vi "GetParam.vi"(8 "error in (no error)":errorcluster caption="entrée d'erreur (pas d'erreur)", 11 "Balanced_Accuracy_Score.lvclass":refnum<class "Balanced_Accuracy_Score.lvclass">) -> (0 "error out":errorcluster caption="sortie d'erreur", 2 "balanced_accuracy_score":cluster{"sample_weight":dbl[], "adjusted":bool}, 3 "Balanced_Accuracy_Score.lvclass":refnum<class "Balanced_Accuracy_Score.lvclass">)   [LabVIEW 2020, in "Balanced_Accuracy_Score.lvclass"]
doc: "Get Parameters"
uses:
  Balanced_Accuracy_Score.lvclass
  Balanced_Accuracy_Score.lvclass/Balanced_Accuracy_Score.ctl
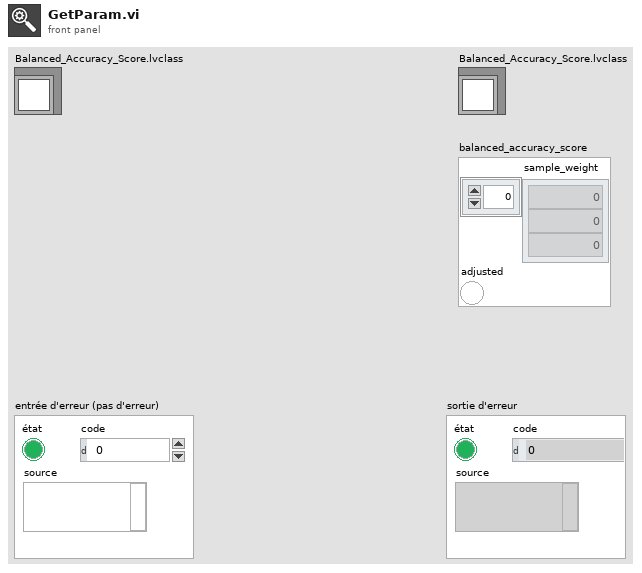
[diagram p1: front panel]
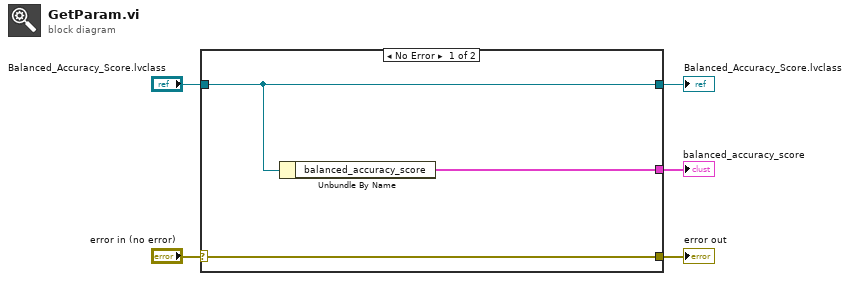
[diagram p0: block diagram]
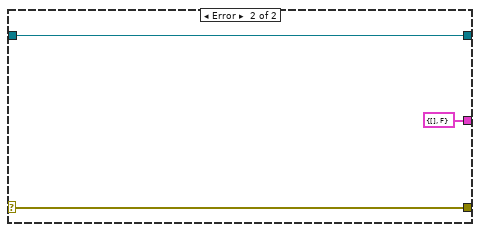
[diagram p2: hidden frame]
diagram:
  n1 = case shown="No Error" "error in (no error)" {
    selector: "error in (no error)" -> [w8 w10]
    tunnel: [w8 w10] -> w4
    tunnel: [w7 w11] -> w2
    tunnel: "Balanced_Accuracy_Score.lvclass" -> [w7 w11]
    tunnel: [w6 cluster{"sample_weight":dbl[], "adjusted":bool} {"sample_weight"=[], "adjusted"=FALSE} ("balanced_accuracy_score")] -> w1
    frame No Error {
      n2 = Unbundle By Name(w7) -> ("balanced_accuracy_score"=w6:cluster{"sample_weight":dbl[], "adjusted":bool})
    }
    frame Error {
    }
  }
  "error out" <- w4
  "Balanced_Accuracy_Score.lvclass" <- w2
  "balanced_accuracy_score" <- w1
